vi "BRig_dataExp_init_setDefault.vi"(11 "input_dataExp":u16[](array[numeric])) -> (3 "output_dataExp":u16[](array[numeric]))   [LabVIEW 2014]
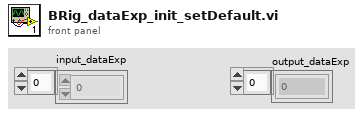
[diagram p1: front panel]
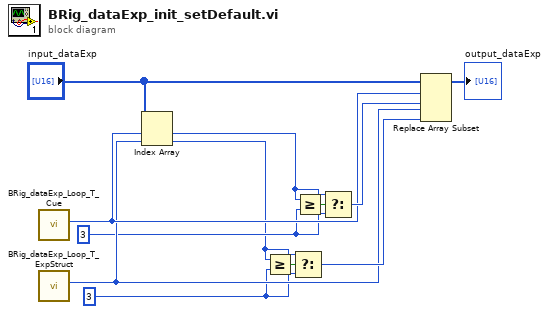
[diagram p0: block diagram]
diagram:
  w1 = u16 3 ("new element/subarray")
  w3 = u16 3 ("new element/subarray")
  n1 = call "BRig_dataExp_Loop_T_Cue.vi"() -> ("output_Loop_T_Cue"=w6:i32)  [unwired: 11 in]
  n2 = call "BRig_dataExp_Loop_T_ExpStruct.vi"() -> ("output_Loop_T_ExpStruct"=w5:i32)  [unwired: 11 in]
  n3 = Index Array(array="input_dataExp", index #1=w6, index #2=w5) -> (element #1=w4:u16, element #2=w2:u16)
  n4 = Greater Or Equal?(x=w2, y=w1) -> (x >= y?=w8:bool)
  n5 = Select(t=w2, s=w8, f=w1) -> (s? t:f=w7:u16)
  n6 = Greater Or Equal?(x=w4, y=w3) -> (x >= y?=w10:bool)
  n7 = Select(t=w4, s=w10, f=w3) -> (s? t:f=w9:u16)
  n8 = Replace Array Subset(array="input_dataExp", new element #1=w9, index #1=w6, new element #2=w7, index #2=w5) -> (→"output_dataExp":u16[])
